vi "Write Status UInt.vi"(4 "error in (no error)":errorcluster, 5 "Status Value":u16 format="%04x", 6 "Status Number":u8=61, 7 "Command":T1(ring)=enum."Set Statuses") -> (0 "error out":errorcluster)   [LabVIEW 2014]
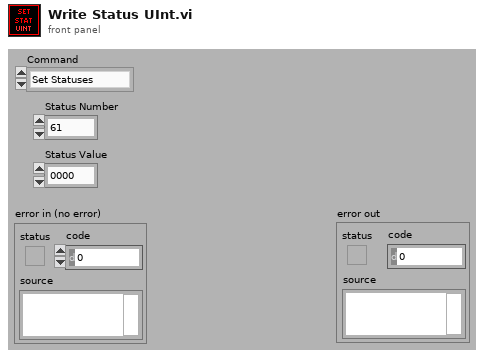
[diagram p1: front panel]
types:
  T1 = enum16{"Default", "Set Statuses", "Set Parameters", "Save Parameter"}
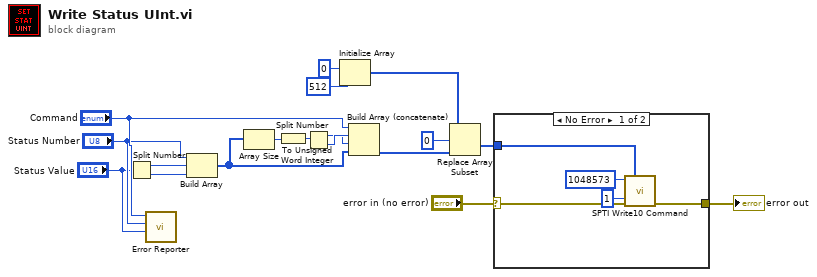
[diagram p0: block diagram]
diagram:
  n1 = Split Number(x="Status Value") -> (hi(x)=w13:u8, lo(x)=w14:u8)
  n2 = call "Error Reporter.vi"("Status Value"="Status Value", "Status Number"="Status Number", "Command"="Command") -> ()  [unwired: 9 in]
  n3 = Build Array("Status Number", w13, w14) -> (w10:u8[])
  n4 = Array Size(array=w10) -> (size(s)=w4:i32)
  n5 = To Unsigned Word Integer(number=w4) -> (unsigned 16bit integer=w5:u16)
  n6 = Split Number(x=w5) -> (hi(x)=w6:u8, lo(x)=w7:u8)
  n7 = Initialize Array(u8 0 ("element"), 512 ("dimension size")) -> (w12:u8[])
  n8 = Build Array (concatenate)("Command", w7, w6, w10) -> (w9:u16[])
  n9 = Replace Array Subset(array=w12, new element=w9, index=0) -> (w11:u8[])
  n10 = case shown="No Error" "error in (no error)" {
    selector: "error in (no error)" -> [w20 w24]
    tunnel: [w21 w24] -> w16
    tunnel: w11 -> [w19 _]
    frame No Error {
      n11 = call "SPTI Write10 Command.vi"("Data to be Written"=w19, "error in (no error)"=w20, "Nr Blocks"=u32 1, "Start LBA"=u32 1048573) -> ("error out"=w21:errorcluster)  [unwired: 6 in, 1 out]
    }
    frame Error {
    }
  }
  "error out" <- w16
